vi "SeqAnalyzeImage.vi"(0 "Color":u32(colorbox)=16711680, 5 "Script Path":string, 7 "Index":i32, 9 "coordinate space":bool, 11 "error in":errorcluster, 12 "CreatDllImage":bool, 13 "Cam Index":i32) -> (4 "VarName":string, 6 "Description":string, 8 "Criteria":string[](array[string]), 10 "data string":string, 14 "return":i32, 15 "error out":errorcluster)   [LabVIEW 2019]
uses:
  ROI/Controls/ROI_List_Action.ctl
  [Global] ItemNames.vi
  [Global] RootPath.vi
  Analysis/Controls/Analysis_Result_To_Caliper.ctl
  Caliper/Controls/Caliper_Entry_FGV_Action.ctl
  Caliper/Controls/AnalysisResultPointsAction.ctl
  [Global] Image Overlay.vi
  [Global] Image.vi
  Controls/Parameter.ctl
  <vilib>/vision/NI_Vision_Development_Module.lvlib
  [Global]CalTemp.vi
  [Global] Template.vi
  Coordinate/Control/CoordinateAction.ctl
panel:
  in  "Script Index":i32
  out "DataValues":dbl[](array[numeric])
  out "TableValues":string[](array[string])
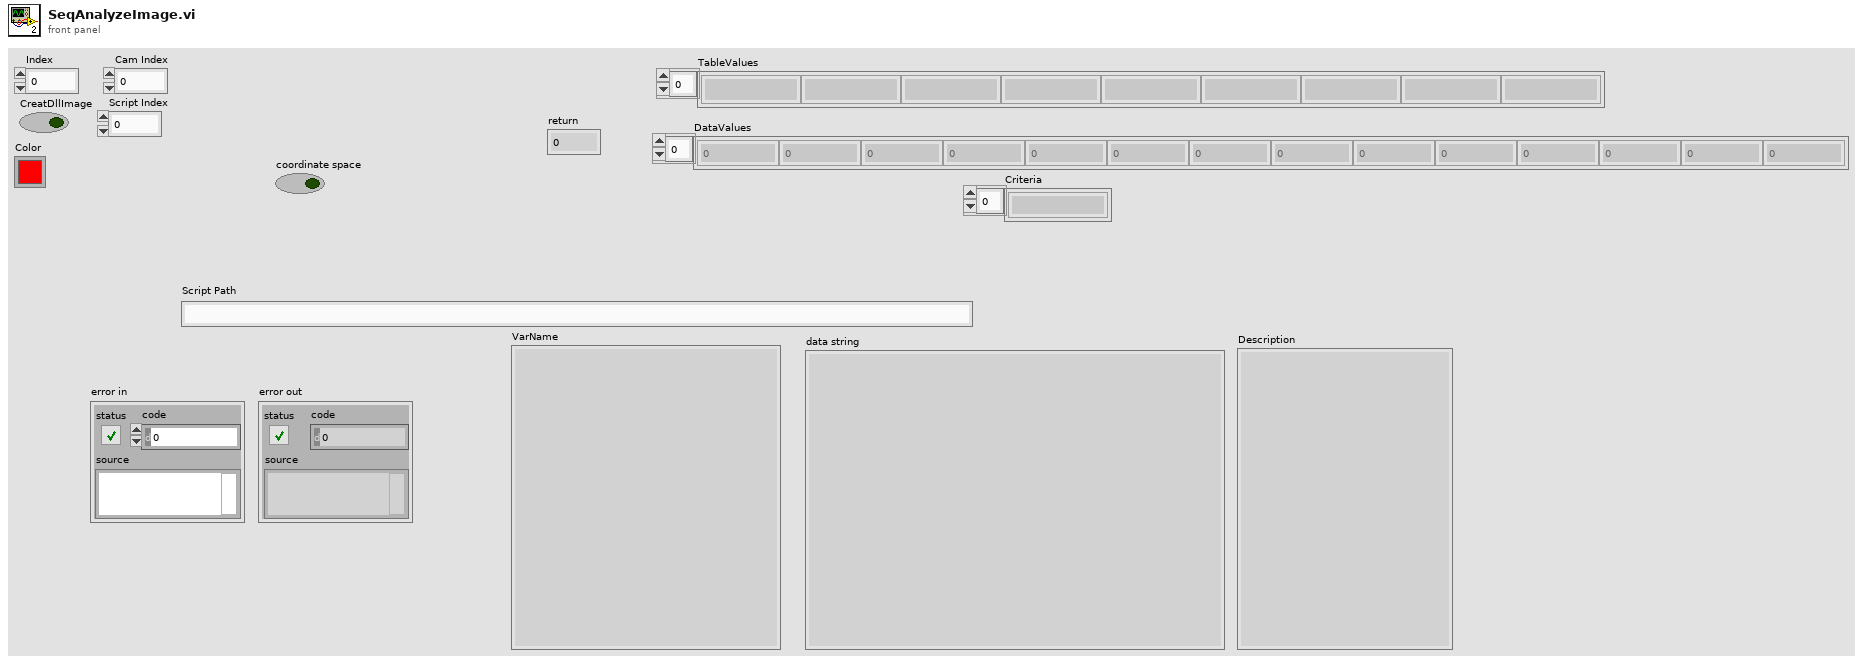
[diagram p1: front panel]
types:
  T1 = enum16{"Init", "Add", "Remove", "Read All", "Remove All", "WriteCriteria"}
  T2 = typedef "CoordinateAction.ctl" = enum16{"Initialize", "CoordEntryInput", "CoordEntryOutput", "CoordEntryTemp", "CoordEntryBackup", "CoordEntryReturn"}
  T3 = typedef "Parameter.ctl" = enum16{"Initialize", "Write", "Read", "WriteAll", "Save", "Load"}
  T4 = typedef "ROI_List_Action.ctl" = enum16{"Init", "Add ROI", "Delete ROI", "Get All ROI", "Get Specific ROI", "Set Analysis Setting", "Set Process Setting", "Replace All Entries", "ROIEntryBackup", "ROIEntryBackupClear", "ROIEntryReturn"}
  T5 = typedef "Caliper_Entry_FGV_Action.ctl" = enum16{"Init", "Close", "Add", "Delete", "ReplaceAll", "ReadAll"}
  T6 = typedef "AnalysisResultPointsAction.ctl" = enum16{"Init", "Add", "Delete", "ReplaceAll", "ReadAll", "Close"}
  T7 = typedef "IMAQ Image.ctl" = refnum<image>
  T8 = typedef "ParameterData.ctl" = cluster{"Rotate Angle":dbl, "Rotate?":bool, "Calibration File Path":string, "Cal?":bool}
  T9 = cluster{"Script Name":string, "TemplateArray":cluster{"ROI Name":string, "TemplateImage":T7}[]}[]
  T10 = typedef "CoordinatteEntry.ctl" = cluster{"ProcessSetting":T11[], "Project Name":string, "AnalysisSetting":T13[], "Coord?":bool, "OriginPointInfo":cluster{"Output Original":bool, "Origin Name":string, "Angle":dbl, "Mode":u16, "OriginPoint":cluster{"X":dbl, "Y":dbl}}, "CaliperSetting":T15[], "CoordIndex":i32[]}
  T11 = typedef "Process_Setting.ctl" = cluster{"Enum_PreProcess":T12, "Parameter":string}
  T12 = typedef "VisionProcessName.ctl" = enum16{"*CamParameter*", "CamAttributes", "*Preprocess*", "CG_Brightness", "C_Plane Extraction", "C_Threshold", "G_Lookup Table", "G_Threshold", "B_Image Inversion"}
  T13 = typedef "CoordinateAnalysisSetting.ctl" = cluster{"Analysis_Type":enum16{"PatternMatch", "Straight Edge"}, "ROI ":T14, "Parameter":variant, "Step Result":variant, "AnalysisStepName":string, "CoordinateUse":bool}
  T14 = typedef "ROI Descriptor" = cluster{"Global Rectangle":i32[], "Contours":cluster{"ID":enum32{"External", "Internal"}, "Type":u32, "Coordinates":i32[]}[]}
  T15 = typedef "CoordinateCaliperSetting.ctl" = cluster{"Result":variant, "CoordinateUse":bool, "CaliperEntry":T16}
  T16 = typedef "CaliperDataEntry.ctl" = cluster{"CaliperType":T17, "Points":T18[], "Result":T20, "StepName":string}
  T17 = typedef "CaliperType.ctl" = u32
  T18 = typedef "SelectionListEntry.ctl" = cluster{"Type":T19, "Index":i32}
  T19 = typedef "SelectionListEntryPointType.ctl" = enum16{"AnalysisResult", "CaliperResult"}
  T20 = typedef "CaliperResult.ctl" = cluster{"PointInclude?":bool, "Num_Of_Pts":u8, "Position.X":dbl, "Position.Y":dbl, "Angle":dbl, "Distance":dbl, "Area":dbl, "Radius_MAX":dbl, "Radius2_min":dbl, "Dev_Residual":dbl, "P2.X":dbl, "P2.Y":dbl, "StepName":string, "Point ID":u8, "StepError?":bool, "ResultDiff?":bool}
  T21 = typedef "IMAQ Coordinate System" = cluster{"Reference System":cluster{"Origin":cluster{"X":sgl, "Y":sgl}, "Angle (deg)":sgl, "Axis Reference":u32}, "Measurement System":cluster{"Origin":cluster{"X":sgl, "Y":sgl}, "Angle (deg)":sgl, "Axis Reference":u32}}
  T22 = typedef "Vision_DataEntry.ctl" = cluster{"vROIName":string, "vROIContour":cluster{"Contour Type":u32, "ROI Type":u32, "Points":i32[]}, "ProcessSetting":T11[], "Analysis_Setting":T23}
  T23 = typedef "Analysis_Setting.ctl" = cluster{"PreProcess":T24, "Parameter":string}
  T24 = typedef "V_Analysis_Type.ctl" = enum16{"None", "C_Color Pattern Matching", "G_PatternMatching", "G_ShapeDectect"}
  T25 = typedef "Analysis_Result_To_Caliper.ctl" = cluster{"PointName":string, "Position_X":dbl, "Position_Y":dbl}
  T26 = cluster{"OutputList":u16[], "Criteria Condition":string[]}
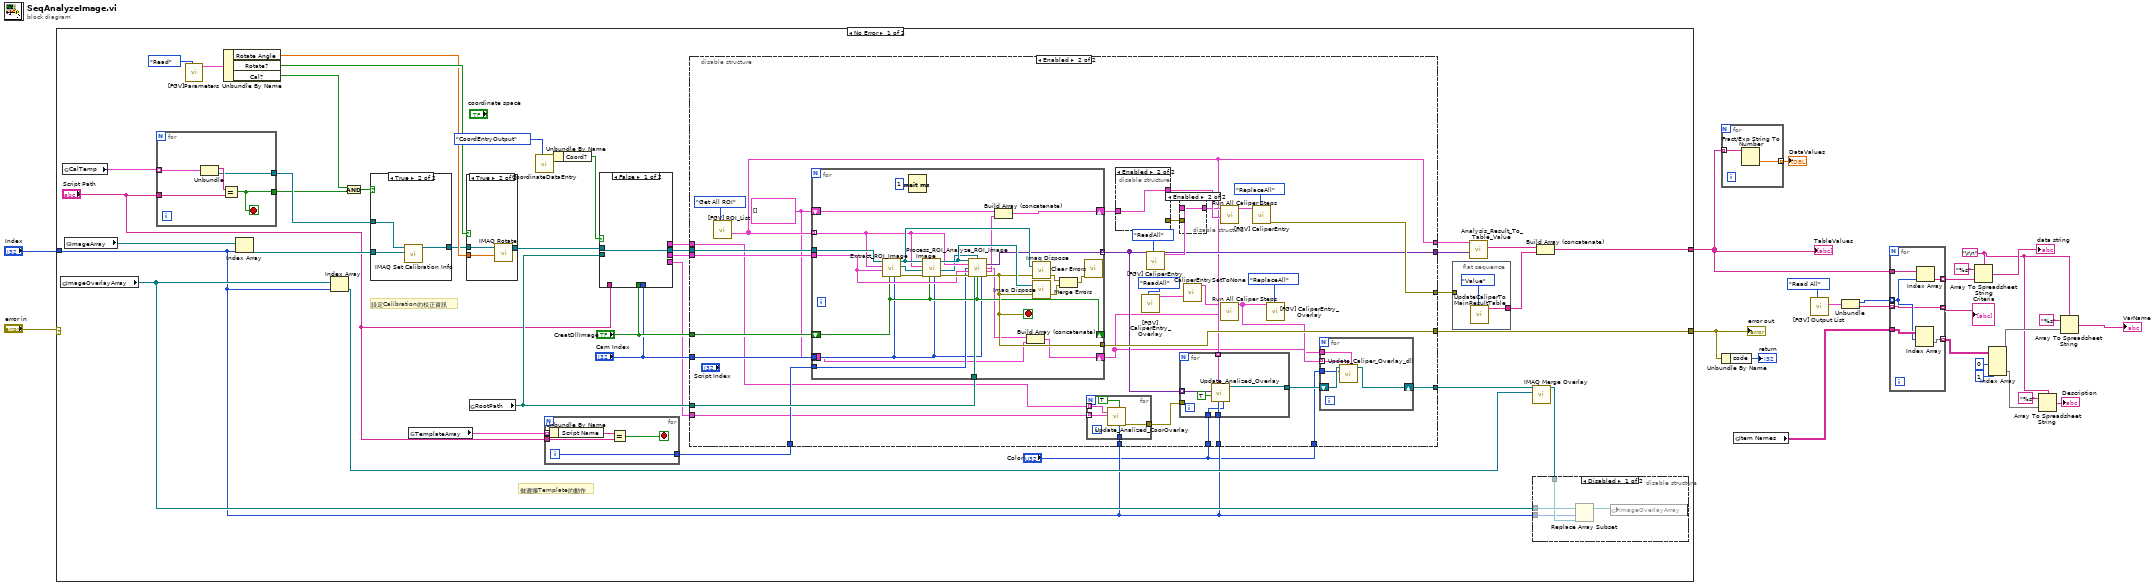
[diagram p0: block diagram]
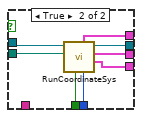
[diagram p5: hidden frame]
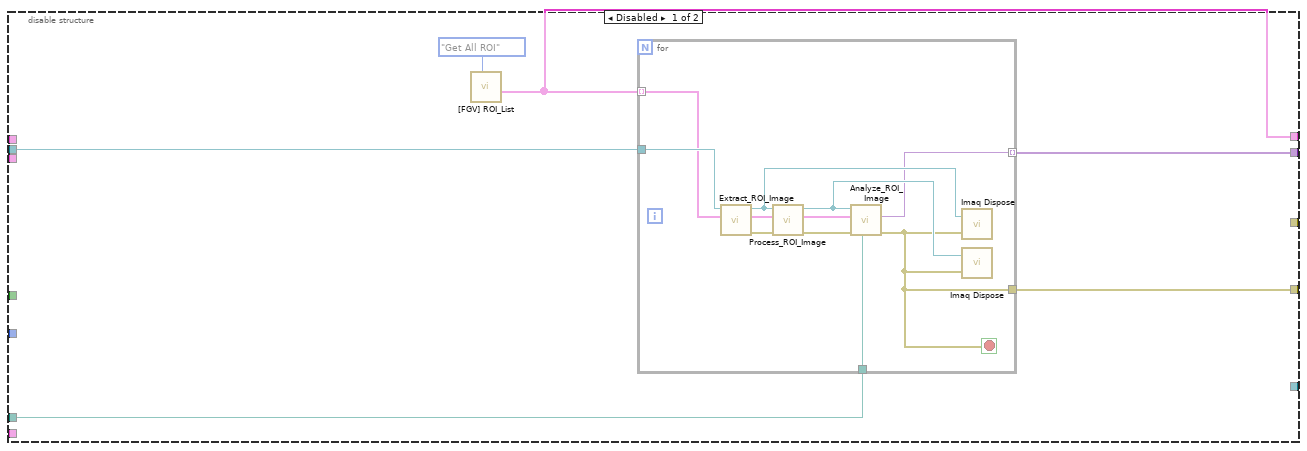
[diagram p6: hidden frame]
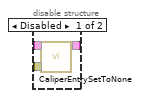
[diagram p7: hidden frame]
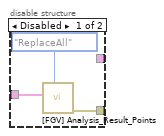
[diagram p8: hidden frame]
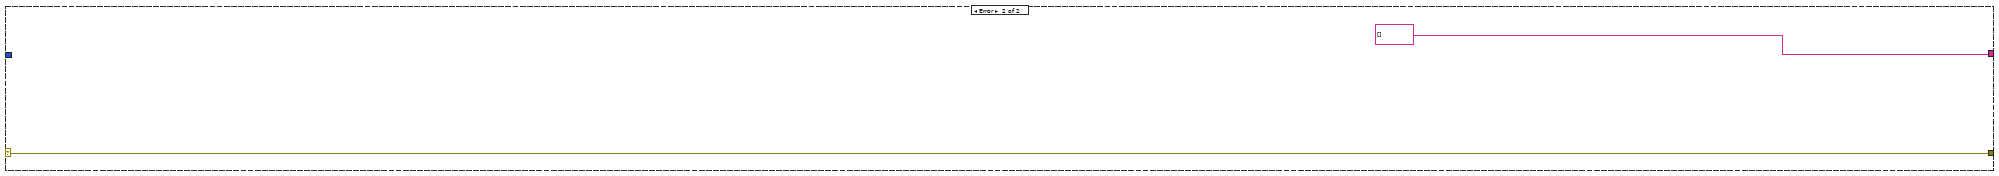
[diagram p9: hidden frame]
diagram:
  w6 = "\r\n"
  n1 = case shown="No Error" "error in" {
    selector: "error in" -> [_ w198]
    tunnel: [w59 string[] [] ("TableValues")] -> w11
    tunnel: [w64 w198] -> w24
    tunnel: "Index" -> [w29 _]
    frame No Error {
      # "做選擇Template的動作"
      # "設定Calibration的校正資訊"
      n2 = global read "[Global] Image Overlay.vi" "ImageOverlayArray"() -> (w51:T7[])
      n3 = global read "[Global]CalTemp.vi" "CalTemp"() -> (w39:cluster{"Script Name":string, "CalImage":T7}[])
      n4 = global read "[Global] Image.vi" "ImageArray"() -> (w53:T7[])
      n5 = for {
        tunnel: w39 -> [w74] mode=indexing
        tunnel: "Script Path" -> [w72]
        tunnel: [w71] -> w38
        tunnel: [w70] -> w36
        stop <- w70 stop-if-true
        n6 = Unbundle(w74) -> ("Script Name"=w73:string, "CalImage"=w71:T7)
        n7 = Equal?(x=w73, y=w72) -> (x = y?=w70:bool)
      }
      n8 = call "[FGV]Parameters.vi"("Parameter"=Parameter."Read") -> ("ParameterData Out"=w46:T8)  [unwired: 9 in, 1 out]
      n9 = Unbundle By Name(w46) -> ("Rotate Angle"=w43:dbl, "Rotate?"=w44:bool, "Cal?"=w41:bool)
      n10 = Index Array(array=w53, index=w29) -> (element=w42:T7)
      n11 = Index Array(array=w51, index=w29) -> (element=w52:T7)
      n12 = And(x=w41, y=w36) -> (x .and. y?=w37:bool)
      n13 = case shown="True" w37 {
        tunnel: w42 -> [w75 w78]
        tunnel: [w75 w77] -> w40
        tunnel: w38 -> [_ w76]
        frame False {
        }
        frame True {
          n14 = call "IMAQ Set Calibration Info"("Image Dst"=w78, "Image Src"=w76) -> ("Calibrated Image"=w77:T7)  [unwired: 2 in, 7 out]
        }
      }
      n15 = global read "[Global] Template.vi" "TemplateArray"() -> (w35:T9)
      n16 = case shown="True" w44 {
        tunnel: w40 -> [w79 w82]
        tunnel: [w79 w81] -> w45
        tunnel: w43 -> [_ w80]
        frame False {
        }
        frame True {
          n17 = call "IMAQ Rotate"("Angle (degrees)"=w80, "Image Src"=w82) -> ("Image Dst Out"=w81:T7)  [unwired: 8 in, 1 out]
        }
      }
      n18 = global read "[Global] RootPath.vi" "RootPath"() -> (w54:path)
      n19 = call "CoordinateDataEntry.vi"("CoordinateAction"=CoordinateAction."CoordEntryOutput") -> ("CoordinatteEntry Output"=w32:T10)  [unwired: 9 in, 1 out]
      n20 = for {
        tunnel: w35 -> [w69] mode=indexing
        tunnel: "Script Path" -> [w67]
        tunnel: [w65] -> w34
        i -> [w65]
        stop <- w66 stop-if-true
        n21 = Unbundle By Name(w69) -> ("Script Name"=w68:string)
        n22 = Equal?(x=w68, y=w67) -> (x = y?=w66:bool)
      }
      n23 = Unbundle By Name(w32) -> ("Coord?"=w31:bool)
      n24 = case shown="False" w31 {
        tunnel: w45 -> [w87 w95]
        tunnel: [w87 w94] -> w56
        tunnel: [_ w93] -> w55
        tunnel: w54 -> [_ w92]
        tunnel: "CreatDllImage" -> [_ w91]
        tunnel: "Cam Index" -> [_ w90]
        tunnel: "Script Path" -> [_ _]
        tunnel: [_ w89] -> w28
        tunnel: [_ w88] -> w27
        frame False {
        }
        frame True {
          n25 = call "RunCoordinateSys.vi"("Dllindex"=w90, "CreatDllImage"=w91, "RootPath"=w92, "Image In"=w95) -> ("AnalysisSetting"=w89:T13[], "Coordinate System Out"=w93:T21, "Vision_Image Out"=w94:T7, "Main Out"=w88:T22[])  [unwired: 3 in, 1 out]
        }
      }
      n26 = disable-structure shown="Enabled" {
        disable-tunnel: [w103 w136] -> w64
        disable-tunnel: w56 -> [w102 w130]
        disable-tunnel: [w100 w135] -> w63
        disable-tunnel: [w99 w134] -> w62
        disable-tunnel: w54 -> [w98 w138]
        disable-tunnel: [_ w137] -> w58
        disable-tunnel: [_ w115] -> w57
        disable-tunnel: w55 -> [_ w133]
        disable-tunnel: "CreatDllImage" -> [_ w132]
        disable-tunnel: "Cam Index" -> [_ w131]
        disable-tunnel: w29 -> [_ w129]
        disable-tunnel: w34 -> [_ w128]
        disable-tunnel: w29 -> [_ w127]
        disable-tunnel: w28 -> [_ w126]
        disable-tunnel: w27 -> [_ w125]
        disable-tunnel: "Color" -> [_ w114]
        disable-tunnel: "Color" -> [_ w113]
        frame Disabled {
          n27 = call "[FGV] ROI_List.vi"("Action"=ROI_List_Action."Get All ROI") -> ("All ROI"=w99:T22[])  [unwired: 8 in, 2 out]
          n28 = for {
            tunnel: w99 -> [w106] mode=indexing
            tunnel: w102 -> [w111]
            tunnel: [w107] -> w100 mode=indexing
            tunnel: [w105] -> w103
            tunnel: w98 -> [w104]
            stop <- w105 stop-if-true
            n29 = call "Extract_ROI_Image.vi"("ROI Entry"=w106, "ImageIn"=w111) -> ("error out"=w112:errorcluster, "ExtractedOriginalImage"=w109:T7)  [unwired: 7 in, 1 out]
            n30 = call "Process_ROI_Image.vi"("error in (no error)"=w112, "ROI Entry"=w106, "ImageIn"=w109) -> ("error out"=w110:errorcluster, "ExtractedProcessedImage"=w108:T7)  [unwired: 6 in, 1 out]
            n31 = call "Analyze_ROI_Image.vi"("RootPath"=w104, "error in (no error)"=w110, "ROI Entry"=w106, "ImageIn"=w108) -> ("error out"=w105:errorcluster, "AnalysisResult"=w107:variant)  [unwired: 4 in, 2 out]
            n32 = call "Imaq Dispose"("Image"=w109, "error in (no error)"=w105) -> ()  [unwired: 4 in, 1 out]
            n33 = call "Imaq Dispose"("Image"=w108, "error in (no error)"=w105) -> ()  [unwired: 4 in, 1 out]
          }
        }
        frame Enabled {
          w119 = T25[] [] ("Analysis_Point_Result")
          n34 = call "[FGV] ROI_List.vi"("Action"=ROI_List_Action."Get All ROI") -> ("All ROI"=w134:T22[])  [unwired: 8 in, 2 out]
          n35 = for {
            tunnel: w134 -> [w190] mode=indexing
            tunnel: w130 -> [w195]
            tunnel: [w191] -> w135 mode=indexing
            tunnel: w138 -> [w189]
            shift-right: [w186] -> w140
            shift-left: w119 -> [w188]
            tunnel: [w185] -> w136
            tunnel: w133 -> [w184]
            tunnel: w131 -> [w181]
            shift-right: [w183] -> _
            shift-left: w132 -> [w183]
            tunnel: w128 -> [w182]
            shift-right: [w175] -> w117
            shift-left: w119 -> [w177]
            stop <- w185 stop-if-true
            n36 = call "Extract_ROI_Image.vi"("Dllindex"=w181, "CreatDllImage"=w183, "Coordinate System Out"=w184, "ROI Entry"=w190, "ImageIn"=w195) -> ("error out"=w196:errorcluster, "ForCalCalculaton Out"=w179:T7, "ExtractedOriginalImage"=w193:T7)  [unwired: 4 in]
            n37 = Wait (ms)(milliseconds to wait=u32 1) -> ()  [unwired: 1 out]
            n38 = call "Process_ROI_Image.vi"("Dllindex"=w181, "CreatDllImage"=w183, "error in (no error)"=w196, "ForCalCalculaton In"=w179, "ROI Entry"=w190, "ImageIn"=w193) -> ("error out"=w194:errorcluster, "ForCalCalculaton Out"=w178:T7, "ExtractedProcessedImage"=w192:T7)  [unwired: 3 in]
            n39 = call "Analyze_ROI_Image.vi"("ImageIn"=w192, "ForCalCalculaton In"=w178, "ROI Entry"=w190, "Script Index"=w182, "Coordinate System In"=w184, "error in (no error)"=w194, "RootPath"=w189, "CreatDllImage"=w183, "Cam Index"=w181) -> ("AnalysisResult"=w191:variant, "Analysis_Point_Result Out Overlay"=w176:T25[], "Analysis_Point_Result"=w187:T25[], "error out"=w185:errorcluster)  [unwired: 2 in, 1 out]
            n40 = Build Array (concatenate)(w188, w187) -> (w186:T25[])
            n41 = Build Array (concatenate)(w176, w177) -> (w175:T25[])
            n42 = call "Imaq Dispose"("Image"=w193, "error in (no error)"=w185) -> ("error out"=w174:errorcluster)  [unwired: 4 in]
            n43 = call "Imaq Dispose"("Image"=w192, "error in (no error)"=w185) -> ("error out"=w173:errorcluster)  [unwired: 4 in]
            n44 = Merge Errors(w174, w173) -> (w172:errorcluster)
            n45 = call <vilib>:"Clear Errors.vi"("error in (no error)"=w172) -> ()  [unwired: 5 in, 2 out]
          }
          n46 = for {
            tunnel: w127 -> [w157]
            tunnel: w126 -> [w155] mode=indexing
            tunnel: w125 -> [w154] mode=indexing
            tunnel: [w153] -> w124
            n47 = call "Update_Analized_CoorOverlay.vi"("Index"=w157, "DLL/Vision"=TRUE, "ROI Entry"=w154, "AnalysisResult"=w155) -> ("error out"=w153:errorcluster)  [unwired: 6 in, 1 out]
          }
          n48 = disable-structure shown="Enabled" {
            disable-tunnel: w140 -> [w169 w171]
            disable-tunnel: [w168 _] -> w143
            disable-tunnel: [_ w171] -> w145
            frame Disabled {
              n49 = call "[FGV] Analysis_Result_Points.vi"("Action"=AnalysisResultPointsAction."ReplaceAll", "Analysis_Point_Result"=w169) -> ("error out"=w168:errorcluster)  [unwired: 8 in, 1 out]
            }
            frame Enabled {
            }
          }
          n50 = call "[FGV] CaliperEntry_Overlay.vi"("Action"=Caliper_Entry_FGV_Action."ReadAll") -> ("AllCaliperEntries"=w121:T16[])  [unwired: 9 in, 1 out]
          n51 = call "[FGV] CaliperEntry.vi"("Action"=Caliper_Entry_FGV_Action."ReadAll") -> ("AllCaliperEntries"=w144:T16[])  [unwired: 9 in, 1 out]
          n52 = disable-structure shown="Enabled" {
            disable-tunnel: w144 -> [w166 w167]
            disable-tunnel: w143 -> [w165 _]
            disable-tunnel: [w164 w167] -> w141
            frame Disabled {
              n53 = call "CaliperEntrySetToNone.vi"("error in (no error)"=w165, "CaliperEntryList"=w166) -> ("CaliperEntryOut"=w164:T16[])  [unwired: 8 in, 1 out]
            }
            frame Enabled {
            }
          }
          n54 = for {
            tunnel: w135 -> [w163] mode=indexing
            tunnel: w134 -> [w162] mode=indexing
            tunnel: [w161] -> w116
            tunnel: w129 -> [w160]
            tunnel: w124 -> [_]
            tunnel: w114 -> [w158]
            n55 = call "Update_Analized_Overlay.vi"("Color"=w158, "Index"=w160, "ROI Entry"=w162, "DLL/Vision"=TRUE, "AnalysisResult"=w163) -> ("DLL Vision_Image"=w161:T7)  [unwired: 5 in, 1 out]
          }
          n56 = call "CaliperEntrySetToNone.vi"("CaliperEntryList"=w121) -> ("CaliperEntryOut"=w122:T16[])  [unwired: 9 in, 1 out]
          n57 = call "Run All Caliper Steps.vi"("Analysis_Point_Result"=w117, "CaliperEntryList"=w122) -> ("CaliperEntryOut"=w118:T16[])  [unwired: 9 in]
          n58 = call "Run All Caliper Steps.vi"("Analysis_Point_Result"=w145, "CaliperEntryList"=w141) -> ("CaliperEntryOut"=w147:T16[])  [unwired: 9 in]
          n59 = call "[FGV] CaliperEntry.vi"("Action"=Caliper_Entry_FGV_Action."ReplaceAll", "CaliperEntriesIn"=w147) -> ("error out"=w137:errorcluster)  [unwired: 8 in, 1 out]
          n60 = call "[FGV] CaliperEntry_Overlay.vi"("Action"=Caliper_Entry_FGV_Action."ReplaceAll", "CaliperEntriesIn"=w118) -> ()  [unwired: 8 in, 2 out]
          n61 = for {
            tunnel: w118 -> [w152] mode=indexing
            tunnel: w117 -> [w151]
            shift-right: [w149] -> w115
            shift-left: w116 -> [w150]
            tunnel: w113 -> [w148]
            n62 = call "Update_Caliper_Overlay_dll.vi"("Analysis_Point_Result"=w151, "CaliperEntry"=w152, "OverlayColor"=w148, "DLL Vision_Image"=w150) -> ("DLL Vision_Image Out"=w149:T7)  [unwired: 7 in]
          }
        }
      }
      n63 = flat-sequence {
        tunnel: [w96] -> w60
        tunnel: w58 -> [_]
        frame #0 {
          n64 = call "UpdateCaliperToMainResultTable.vi"("Type"=enum16{"TagName", "Value"}."Value") -> ("CaliperResultNames"=w96:string[])  [unwired: 10 in]
        }
      }
      n65 = call "Analysis_Result_To_Table_Value.vi"("AnalysisResults"=w63, "All ROI"=w62) -> ("TableValues"=w61:string[])  [unwired: 9 in]
      n66 = call "IMAQ Merge Overlay"("Image Dst"=w52, "Image Src"=w57) -> ("Image Dst Out"=w50:T7)  [unwired: 8 in, 1 out]
      n67 = disable-structure shown="Disabled" {
        disable-tunnel: w51 -> [w86 _]
        disable-tunnel: w50 -> [w85 _]
        disable-tunnel: w29 -> [w83 _]
        frame Disabled {
          n68 = Replace Array Subset(array=w86, new element=w85, index=w83) -> (w84:T7[])
          n69 = global write "[Global] Image Overlay.vi" "ImageOverlayArray"(w84) -> ()
        }
        frame Enabled {
        }
      }
      n70 = Build Array (concatenate)(w61, w60) -> (w59:string[])
    }
    frame Error {
    }
  }
  "TableValues" <- w11
  "error out" <- w24
  n71 = for {
    tunnel: w11 -> [w200] mode=indexing
    tunnel: [w199] -> w22 mode=indexing
    n72 = Fract/Exp String To Number(string=w200) -> (number=w199:dbl)  [unwired: 3 in, 1 out]
  }
  "DataValues" <- w22
  n73 = Unbundle By Name(w24) -> ("code"=→"return":i32)
  n74 = global read "[Global] ItemNames.vi" "Item Names"() -> (w8:string[][])
  n75 = call "[FGV] Output List.vi"("Action"=T1."Read All") -> ("Output"=w4:T26)  [unwired: 9 in, 1 out]
  n76 = Unbundle(w4) -> ("OutputList"=w3:u16[], "Criteria Condition"=w2:string[])
  n77 = for {
    tunnel: w2 -> [w201] mode=indexing
    tunnel: w11 -> [w206]
    tunnel: [w205] -> w10 mode=indexing
    tunnel: w8 -> [w204]
    tunnel: [w203] -> w7 mode=indexing
    tunnel: w3 -> [w202] mode=indexing
    tunnel: [w201] -> w1 mode=indexing
    n78 = Index Array(array=w204, index (row)=w202) -> (element=w203:string[])  [unwired: 1 in]
    n79 = Index Array(array=w206, index=w202) -> (element=w205:string)
  }
  "Criteria" <- w1
  n80 = Array To Spreadsheet String(delimiter (Tab)=w6, array=w10, 3:"%s" ("format string")) -> (spreadsheet string=→"data string":string)
  n81 = Index Array(array=w7, index (col) #1=0 ("disabled index (col)"), index (col) #2=1 ("index (col)")) -> (element #1=w18:string[], element #2=w16:string[])  [unwired: 2 in]
  n82 = Array To Spreadsheet String(delimiter (Tab)=w6, array=w16, 3:"%s" ("format string")) -> (spreadsheet string=→"Description":string)
  n83 = Array To Spreadsheet String(delimiter (Tab)=w6, array=w18, 3:"%s" ("format string")) -> (spreadsheet string=→"VarName":string)
